vi "Wait.vi"(6 "milliseconds to wait":u32=20, 8 "error in (no error)":errorcluster, 11 "refnum in":refnum<visa-resource-name>) -> (0 "error out":errorcluster, 3 "refnum out":refnum<visa-resource-name>)   [LabVIEW 2020, in "Korad KA3305P.lvlib"]
uses:
  Korad KA3305P.lvlib
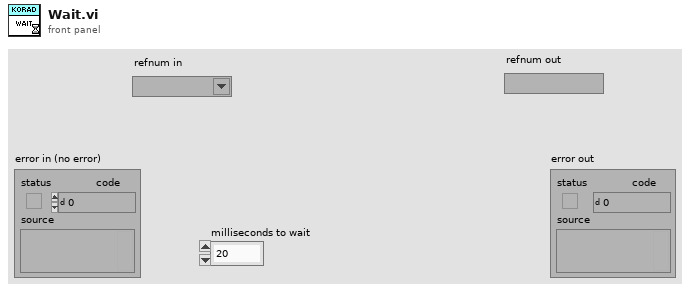
[diagram p1: front panel]
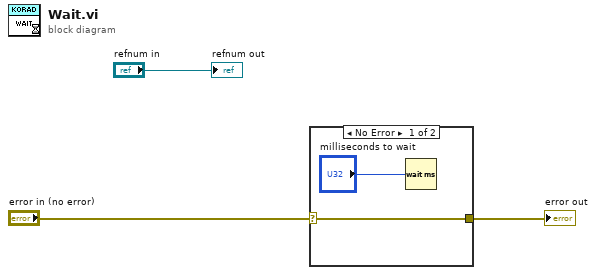
[diagram p0: block diagram]
diagram:
  n1 = case shown="No Error" "error in (no error)" {
    selector: "error in (no error)" -> [w5 w6]
    tunnel: [w5 w6] -> w1
    frame No Error {
      n2 = Wait (ms)(milliseconds to wait="milliseconds to wait") -> ()  [unwired: 1 out]
    }
    frame Error {
    }
  }
  "error out" <- w1
  "refnum out" <- "refnum in"
